vi "Config Cable.vi"(6 "Capacitance (100.0 pF/m)":dbl=100.0 min=0.0 max=999.9 step=0.1 format="%.1f", 7 "Length (1.00 m)":dbl=1.0 min=0.0 max=999.99 step=0.01 format="%.2f", 8 "error in":errorcluster, 9 "Inductance (1.10 microhenry/m)":dbl=1.1 min=0.0 max=99.99 step=0.01 format="%.2f", 10 "Resistance (40.0 milliohm/m)":dbl=40.0 min=0.0 max=9999.0 step=0.1 format="%.1f", 11 "VISA resource name":refnum<visa-resource-name>) -> (0 "error out":errorcluster, 3 "VISA resource name out":refnum<visa-resource-name>)   [LabVIEW 2016, in "Andeen-Hagerling 2550.lvlib"]
doc: "This VI compensates for the characteristics of longer cables or cables used to connect the bridge to larger capacitances."
uses:
  Andeen-Hagerling 2550.lvlib
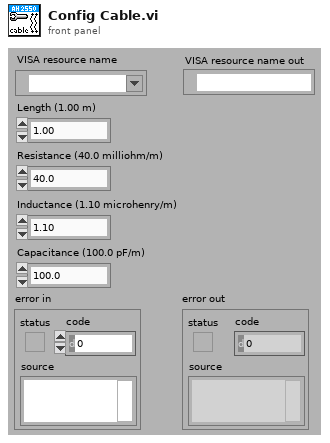
[diagram p1: front panel]
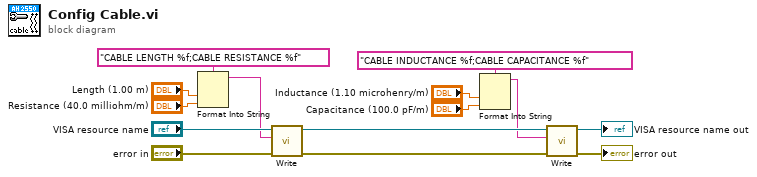
[diagram p0: block diagram]
diagram:
  n1 = Format Into String(format string="CABLE LENGTH %f;CABLE RESISTANCE %f", "Length (1.00 m)", "Resistance (40.0 milliohm/m)") -> (resulting string=w10:string)  [unwired: 2 in, 1 out]
  n2 = call "Write.vi"("error in"="error in", "command"=w10, "VISA resource name"="VISA resource name") -> ("error out"=w6:errorcluster, "VISA resource name out"=w8:refnum<visa-resource-name>)  [unwired: 7 in]
  n3 = Format Into String(format string="CABLE INDUCTANCE %f;CABLE CAPACITANCE %f", "Inductance (1.10 microhenry/m)", "Capacitance (100.0 pF/m)") -> (resulting string=w1:string)  [unwired: 2 in, 1 out]
  n4 = call "Write.vi"("error in"=w6, "command"=w1, "VISA resource name"=w8) -> ("error out"=→"error out":errorcluster, "VISA resource name out"=→"VISA resource name out":refnum<visa-resource-name>)  [unwired: 7 in]
